vi "5三点法.vi"(1 "波形":waveform(dbl)) -> (0 "f":dbl)   [LabVIEW 2017]
uses:
  <vilib>/Analysis/NI_AALPro.lvlib
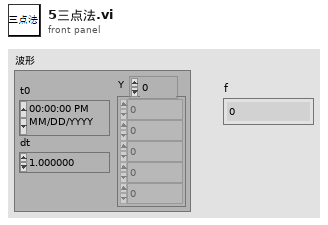
[diagram p1: front panel]
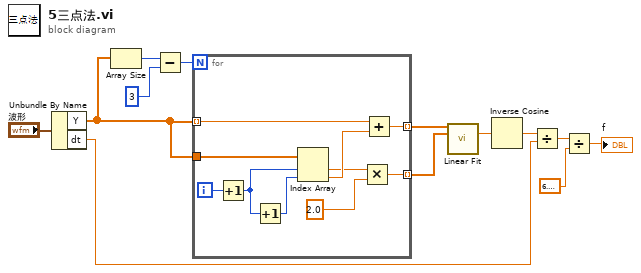
[diagram p0: block diagram]
diagram:
  n1 = Unbundle By Name("波形") -> ("Y"=w12:dbl[], "dt"=w4:dbl)
  n2 = Array Size(array=w12) -> (size(s)=w11:i32)
  n3 = Subtract(x=w11, y=3) -> (x-y=w9:i32)
  n4 = for {
    N: w9 -> [_]
    tunnel: w12 -> [w19] mode=indexing
    tunnel: w12 -> [w23]
    tunnel: [w17] -> w8 mode=indexing
    tunnel: [w15] -> w7 mode=indexing
    i -> [w22]
    n5 = Increment(x=w22) -> (x+1=w21:i32)
    n6 = Increment(x=w21) -> (x+1=w20:i32)
    n7 = Index Array(array=w23, index #1=w21, index #2=w20) -> (element #1=w16:dbl, element #2=w18:dbl)
    n8 = Multiply(x=w16, y=2.0) -> (x*y=w15:dbl)
    n9 = Add(x=w19, y=w18) -> (x+y=w17:dbl)
  }
  n10 = call <vilib>:"Linear Fit.vi"("Y"=w8, "X"=w7) -> ("slope"=w6:dbl)  [unwired: 9 in, 4 out]
  n11 = Inverse Cosine(1:w6) -> (0:w5:dbl)
  n12 = Divide(x=w5, y=w4) -> (x/y=w2:dbl)
  n13 = Divide(x=w2, y=6.283185307179586) -> (x/y=→"f":dbl)
